vi "Write Serial port.vi"(8 "error in (no error)":errorcluster, 10 "Serial port":refnum<visa-resource-name>, 11 "Motor-Serial in":refnum<class "Motor-Serial.lvclass">) -> (0 "error out":errorcluster, 3 "Motor-Serial out":refnum<class "Motor-Serial.lvclass">)   [LabVIEW 2013, in "PowderDeposition.lvlib" / "Motor-Serial.lvclass"]
uses:
  Motor-Serial.lvclass
  Motor-Serial.lvclass/Motor-Serial.ctl
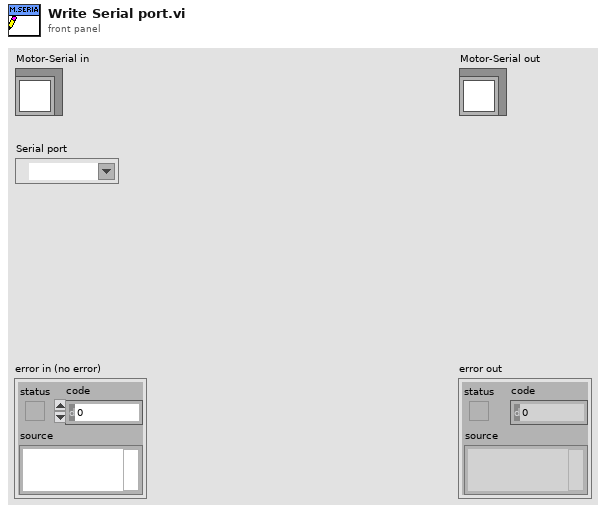
[diagram p1: front panel]
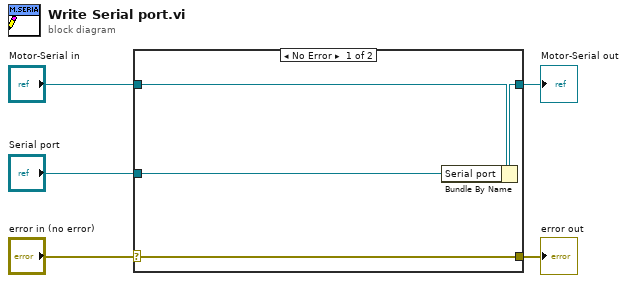
[diagram p0: block diagram]
diagram:
  n1 = case shown="No Error" "error in (no error)" {
    selector: "error in (no error)" -> [w9 w10]
    tunnel: [w9 w10] -> w4
    tunnel: [w7 w11] -> w2
    tunnel: "Motor-Serial in" -> [w8 w11]
    tunnel: "Serial port" -> [w6 _]
    frame No Error {
      n2 = Bundle By Name(cluster=w8, "Serial port"=w6) -> (w7:refnum<class "Motor-Serial.lvclass">)
    }
    frame Error {
    }
  }
  "error out" <- w4
  "Motor-Serial out" <- w2
